vi "FTW-Package-Interpret.vi"(0 "FTW-Message-Lossy In":refnum<class "FTW-Package-Lossy.lvclass">, 11 "error in":errorcluster) -> (4 "FTW-Message-Lossy Out":refnum<class "FTW-Package-Lossy.lvclass">, 6 "Sender Identity":string, 8 "Message Header":string, 10 "Message Body":string, 15 "error out":errorcluster)   [LabVIEW 2013, in "FTW-Package-Lossy.lvclass"]
uses:
  FTW-Package-Lossy.lvclass
panel:
  # "Inputs"
  # "Outputs"
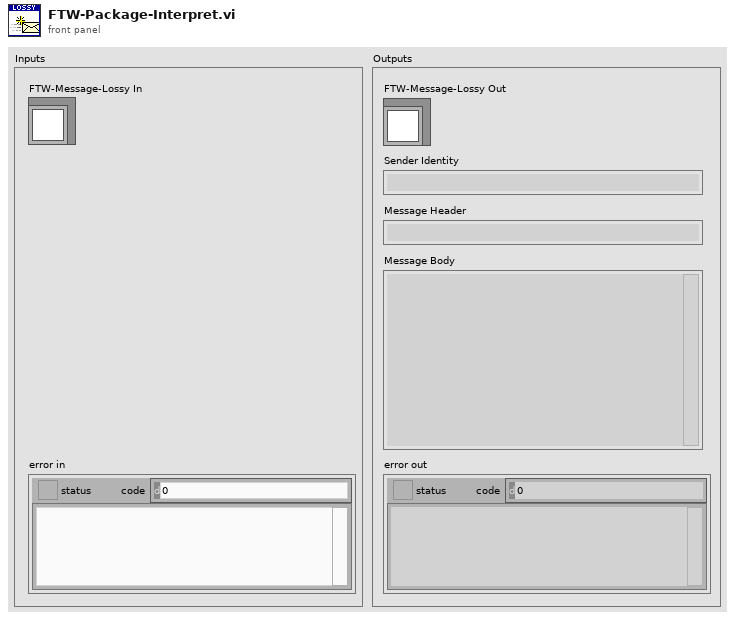
[diagram p1: front panel]
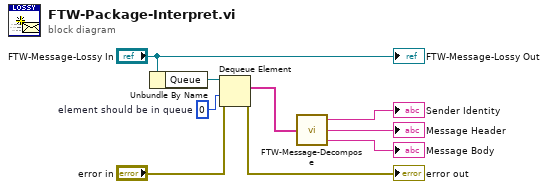
[diagram p0: block diagram]
diagram:
  w1 = 0  # element should be in queue
  n1 = Unbundle By Name("FTW-Message-Lossy In") -> ("Queue"=w5:refnum<queue>)
  n2 = Dequeue Element(queue=w5, timeout in ms (-1)=w1, error in (no error)="error in") -> (element=w4:string[], error out=→"error out":errorcluster)  [unwired: 2 out]
  n3 = call "FTW-Message-Decompose.vi"("Message"=w4) -> ("Sender Identity"=→"Sender Identity":string, "Message Header"=→"Message Header":string, "Message Body"=→"Message Body":string)  [unwired: 1 in]
  "FTW-Message-Lossy Out" <- "FTW-Message-Lossy In"
